vi "PROPORTIONING VALVE DRIVER.vi"(8 "Error In":errorcluster) -> (0 "Error Out":errorcluster)   [LabVIEW 2016]
panel:
  in  "Target":dbl
  in  "MW100 Input":refnum<visa-resource-name>
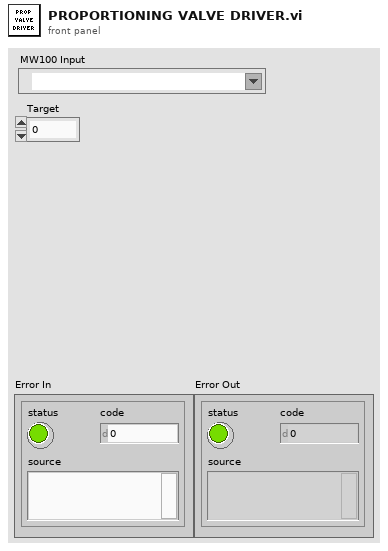
[diagram p1: front panel]
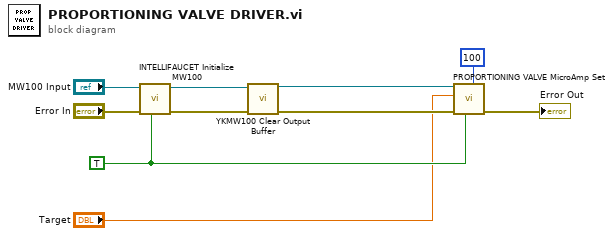
[diagram p0: block diagram]
diagram:
  w4 = TRUE ("Debug")
  n1 = call "INTELLIFAUCET Initialize MW100.vi"("Debug"=w4, "error in (no error)"="Error In", "MW100 Input"="MW100 Input") -> ("error out"=w9:errorcluster, "MW100 Output"=w10:refnum<visa-resource-name>)  [unwired: 6 in, 1 out]
  n2 = call "YKMW100 Clear Output Buffer.vi"("VISA session"=w10, "error in (no error)"=w9) -> ("dup VISA session"=w8:refnum<visa-resource-name>, "error out"=w5:errorcluster)  [unwired: 12 in]
  n3 = call "PROPORTIONING VALVE MicroAmp Set.vi"("milliseconds to wait"=u32 100, "Debug"=w4, "error in (no error)"=w5, "Target"="Target", "VISA Refnum in"=w8) -> ("error out"=→"Error Out":errorcluster)  [unwired: 5 in, 1 out]
